vi "DatabaseHand_Element_Get(I16).vi"(7 "nd queue":bool, 8 "error in (no error)":errorcluster, 9 "default value":i16, 10 "name":string, 11 "Database RefNum in":T1) -> (0 "error out":errorcluster, 1 "type":string, 2 "value":i16, 3 "Database RefNum out":T1, 4 "permissions":string="RW", 5 "group":string, 6 "unit":string)   [LabVIEW 2016]
doc: "This VI finds the RefNum of an existing object with the input Name or creates a new object if the Name is not found or Name is unwired or an empty string.\nCopyright 2001 VI Engineering, Inc."
uses:
  DatabaseHand_RefNum.ctl
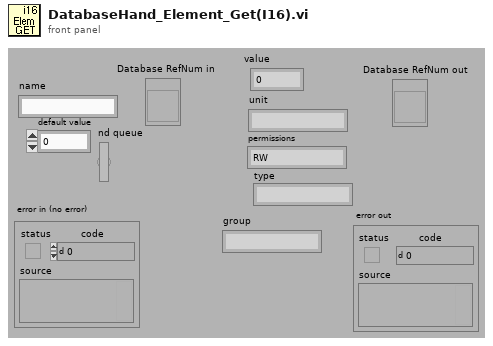
[diagram p1: front panel]
types:
  T1 = typedef "DatabaseHand_RefNum.ctl" = refnum<vi>
  T2 = typedef "DatabaseHand_Element.ctl" = cluster{"name":string, "Database":T3[]}
  T3 = typedef "DatabaseHan_DatabaseElement.ctl" = cluster{"name":string, "value":string, "type":string, "unit":string, "permissions":string, "enqueued":bool, "group":string}
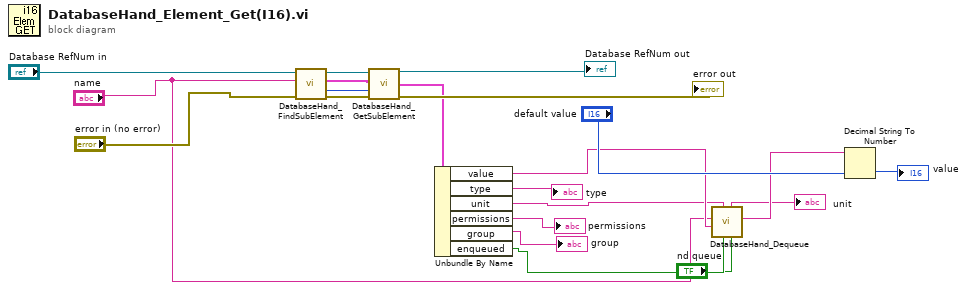
[diagram p0: block diagram]
diagram:
  n1 = call "DatabaseHand_FindSubElement.vi"("error in (no error)"="error in (no error)", "name"="name", "Database RefNum in"="Database RefNum in") -> ("error out"=w17:errorcluster, "index"=w14:i32, "Database"=w18:T2, "Database RefNum out"=w19:T1)  [unwired: 5 out]
  n2 = call "DatabaseHand_GetSubElement.vi"("Database RefNum in"=w19, "Object Data In"=w18, "Index"=w14, "error in (no error)"=w17) -> ("Database RefNum out"=→"Database RefNum out":T1, "Element found"=w13:T3, "error out"=→"error out":errorcluster)  [unwired: 9 out]
  n3 = Unbundle By Name(w13) -> ("value"=w7:string, "type"=→"type":string, "unit"=w2:string, "permissions"=→"permissions":string, "group"=→"group":string, "enqueued"=w4:bool)
  n4 = call "DatabaseHand_Dequeue.vi"("non-destructive queue"="nd queue", "queue?"=w4, "unit in"=w2, "value in"=w7, "name"="name") -> ("value out"=w6:string, "unit out"=→"unit":string)  [unwired: 5 out]
  n5 = Decimal String To Number(string=w6, default (0L)="default value") -> (number=→"value":i16)  [unwired: 2 out]
